vi "Create Test from Class Name.vi"(11 "Test Step":string) -> (3 "Test":refnum<class "Executioner.lvclass">)   [LabVIEW 2019, in "Test Executive.lvlib" / "Executioner.lvclass"]
uses:
  <vilib>/gpm_packages/@cs/test-executive/Source/Test Executive/Executioner/Executioner.lvclass
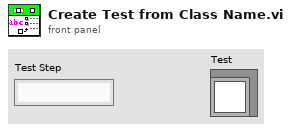
[diagram p1: front panel]
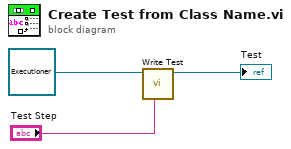
[diagram p0: block diagram]
diagram:
  n1 = call <vilib>:"Write Test.vi"("Test"="Test Step", "Executioner in"=refnum<class "Executioner.lvclass"> refnum ("Test")) -> ("Executioner out"=→"Test":refnum<class "Executioner.lvclass">)  [unwired: 9 in]
